vi "Create Sequence.vi"(0 "VISA Resource Name":refnum<visa-resource-name>, 1 "Sequence Name (SEQUENCE_SEQ)":string="SEQUENCE_SEQ", 2 "Sequence Waveforms":T1(array[cluster]), 5 "error in (no error)":errorcluster {"code" format="%.0x"}) -> (14 "VISA Resource Name Out":refnum<visa-resource-name>, 19 "error out":errorcluster {"code" format="%.0x"})   [LabVIEW 2014, in "Agilent ESG Series.lvlib"]
doc: "This VI creates or defines a waveform sequence. The waveform file consists of the subsequent waveform segment files.\n\nNotes:\n(1) This VI is valid only on instruments Agilent E44xB with the UND option or on instrument E4438C with option 001/601 or 002/602."
uses:
  Agilent ESG Series.lvlib
panel:
  # "TRUE\n\nFALSE"
  # "TRUE\n\nFALSE"
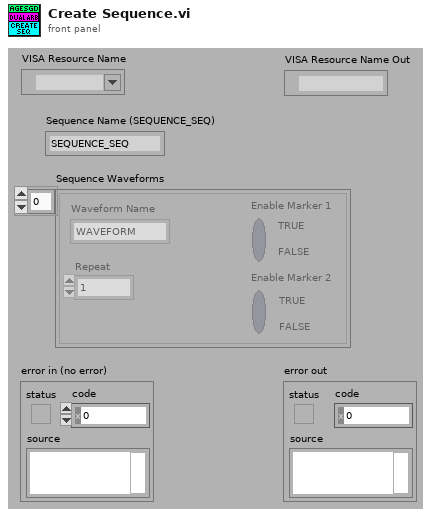
[diagram p1: front panel]
types:
  T1 = cluster{"Waveform Name":string, "Repeat":i32, "Enable Marker 1":bool, "Enable Marker 2":bool}[]
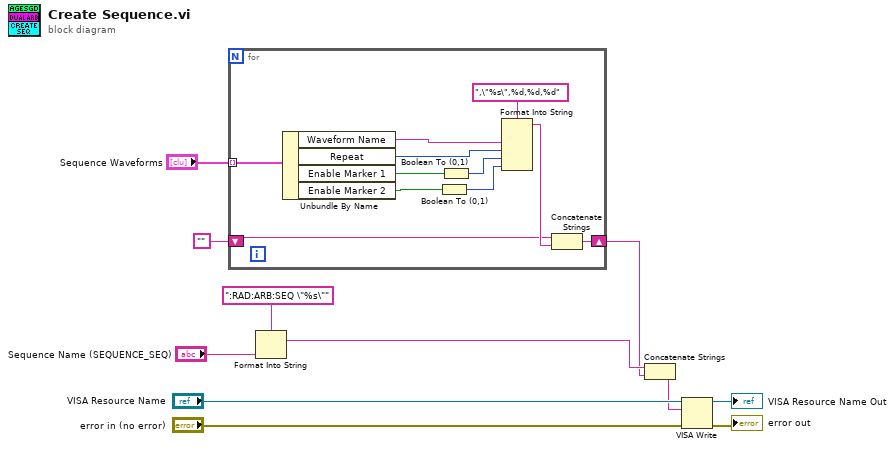
[diagram p0: block diagram]
diagram:
  n1 = for {
    tunnel: "Sequence Waveforms" -> [w21] mode=indexing
    shift-right: [w15] -> w2
    shift-left: "" -> [w12]
    n2 = Unbundle By Name(w21) -> ("Waveform Name"=w14:string, "Repeat"=w20:i32, "Enable Marker 1"=w18:bool, "Enable Marker 2"=w19:bool)
    n3 = Boolean To (0,1)(Boolean=w19) -> (0, 1=w17:i16)
    n4 = Boolean To (0,1)(Boolean=w18) -> (0, 1=w16:i16)
    n5 = Format Into String(format string=",\"%s\",%d,%d,%d", w14, w20, w16, w17) -> (resulting string=w13:string)  [unwired: 2 in, 1 out]
    n6 = Concatenate Strings(w12, w13) -> (w15:string)
  }
  n7 = Format Into String(format string=":RAD:ARB:SEQ \"%s\"", "Sequence Name (SEQUENCE_SEQ)") -> (resulting string=w3:string)  [unwired: 2 in, 1 out]
  n8 = Concatenate Strings(w3, w2) -> (w1:string)
  n9 = VISA Write(VISA resource name="VISA Resource Name", write buffer=w1, error in (no error)="error in (no error)") -> (VISA resource name out=→"VISA Resource Name Out":refnum<visa-resource-name>, error out=→"error out":errorcluster)  [unwired: 1 out]
